vi "CRYLast curve or result read.vi"(8 "Extension":string="Result          ", 11 "Filepath":path) -> (0 "Error":bool, 3 "Flat Data or Result":string)   [LabVIEW 2013]
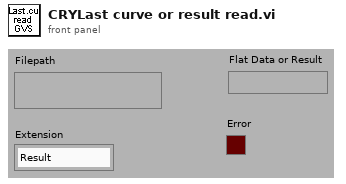
[diagram p1: front panel]
types:
  T1 = enum16{"read/write", "read-only", "write-only", "write-only (truncate)"}
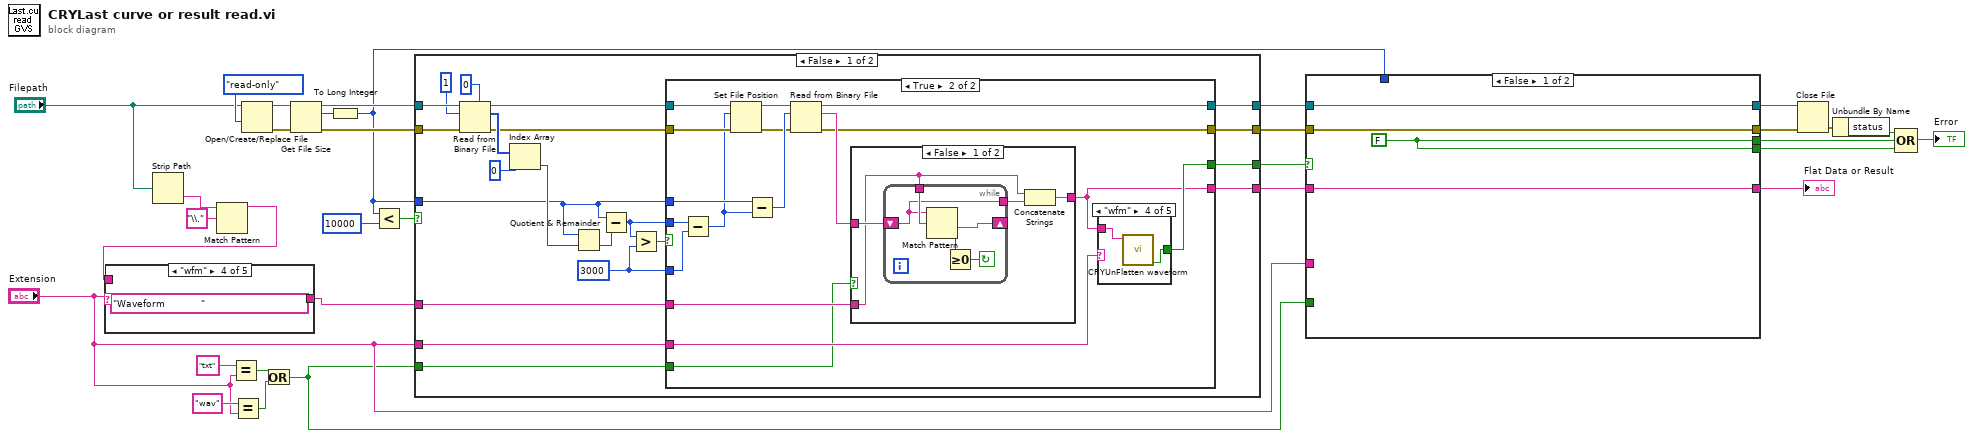
[diagram p0: block diagram]
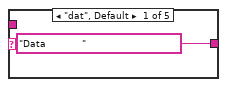
[diagram p2: hidden frame]
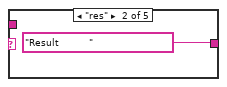
[diagram p3: hidden frame]
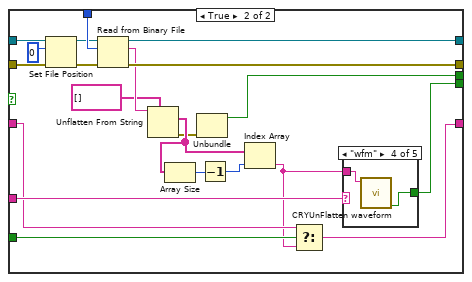
[diagram p6: hidden frame]
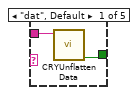
[diagram p7: hidden frame]
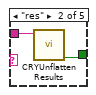
[diagram p8: hidden frame]
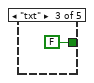
[diagram p9: hidden frame]
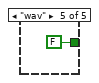
[diagram p10: hidden frame]
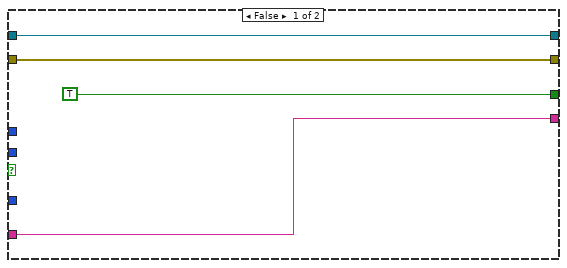
[diagram p11: hidden frame]
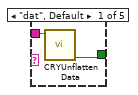
[diagram p13: hidden frame]
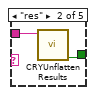
[diagram p14: hidden frame]
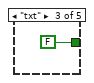
[diagram p15: hidden frame]
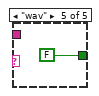
[diagram p16: hidden frame]
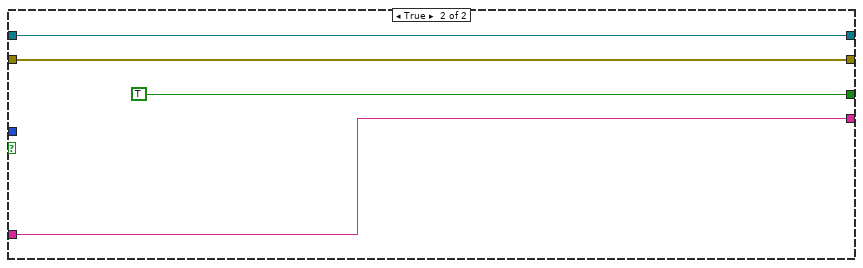
[diagram p17: hidden frame]
diagram:
  n1 = Strip Path(path="Filepath") -> (name=w9:string)  [unwired: 1 out]
  n2 = Match Pattern(string=w9, regular expression="\\.") -> (before substring=w7:string)  [unwired: 1 in, 3 out]
  n3 = case shown="\"wfm\"" "Extension" {
    tunnel: ["Data            " "Result          " w35 "Waveform            " w37] -> w11
    tunnel: w7 -> [_ _ w35 _ w37]
    frame "dat", Default {
    }
    frame "res" {
    }
    frame "txt" {
    }
    frame "wfm" {
    }
    frame "wav" {
    }
  }
  n4 = Equal?(x="txt", y="Extension") -> (x = y?=w5:bool)
  n5 = Equal?(x="wav", y="Extension") -> (x = y?=w6:bool)
  n6 = Open/Create/Replace File(file path (use dialog)="Filepath", access (0:read/write)=T1."read-only" ("open mode (0)")) -> (refnum out=w32:refnum<file>, error out=w31:errorcluster)  [unwired: 1 in, 4 out]
  n7 = Or(x=w5, y=w6) -> (x .or. y?=w1:bool)
  n8 = Get File Size(file=w32, error in=w31) -> (refnum out=w21:refnum<file>, size (in bytes)=w12:i64, 0:w20:errorcluster)
  n9 = To Long Integer(number=w12) -> (32bit integer=w15:i32)
  n10 = Less?(x=w15, y=10000 ("offset")) -> (x < y?=w22:bool)
  n11 = case shown="False" w22 {
    tunnel: w21 -> [w58 w100]
    tunnel: w20 -> [w57 w99]
    tunnel: w15 -> [w41 _]
    tunnel: [w45 TRUE ("Error?")] -> w19
    tunnel: [w44 w98] -> w18
    tunnel: [w43 w99] -> w17
    tunnel: [w42 w100] -> w16
    tunnel: w11 -> [w40 w98]
    tunnel: "Extension" -> [w39 _]
    tunnel: w1 -> [w38 _]
    frame False {
      w48 = 3000 ("y")
      n12 = Read from Binary File(5:0 ("count"), 8:w57, 10:1 ("count"), 11:w58) -> (0:w46:errorcluster, 2:w54:i32[], 3:w47:refnum<file>)  [unwired: 3 out]
      n13 = Index Array(array=w54, index=0 ("Index")) -> (element=w52:i32)
      n14 = Quotient & Remainder(x=w41, y=w52) -> (floor(x/y)=w51:i32)  [unwired: 1 out]
      n15 = Subtract(x=w41, y=w51) -> (x-y=w49:i32)
      n16 = Greater?(x=w49, y=w48) -> (0:w50:bool)
      n17 = case shown="True" w50 {
        tunnel: w49 -> [_ w79]
        tunnel: w48 -> [_ w78]
        tunnel: w47 -> [w61 w77]
        tunnel: w46 -> [w60 w76]
        tunnel: [TRUE ("Error?") w74] -> w45
        tunnel: [w59 w68] -> w44
        tunnel: [w60 w73] -> w43
        tunnel: [w61 w72] -> w42
        tunnel: w41 -> [_ w71]
        tunnel: w40 -> [w59 w67]
        tunnel: w39 -> [_ w64]
        tunnel: w38 -> [_ w63]
        frame False {
        }
        frame True {
          n18 = Subtract(x=w79, y=w78) -> (x-y=w70:i32)
          n19 = Set File Position(offset (in bytes) (0)=w70, refnum=w77, error in=w76) -> (refnum out=w66:refnum<file>, error out=w65:errorcluster)  [unwired: 1 out]
          n20 = Subtract(x=w71, y=w70) -> (x-y=w69:i32)
          n21 = Read from Binary File(8:w65, 10:w69, 11:w66) -> (0:w73:errorcluster, 2:w75:string, 3:w72:refnum<file>)  [unwired: 4 out]
          n22 = case shown="False" w63 {
            tunnel: w75 -> [w83 _]
            tunnel: [w81 w89] -> w68
            tunnel: w67 -> [w80 w89]
            frame False {
              n23 = while {
                tunnel: [w84] -> w82
                tunnel: w80 -> [w88]
                shift-left: w83 -> [w84]
                shift-right: [w87] -> _
                stop <- w85 continue-if-true
                n24 = Match Pattern(string=w84, regular expression=w88) -> (after substring=w87:string, offset past match=w86:i32)  [unwired: 3 out]
                n25 = Greater Or Equal To 0?(x=w86) -> (x >= 0?=w85:bool)
              }
              n26 = Concatenate Strings(w80, w82) -> (w81:string)
            }
            frame True {
            }
          }
          n27 = case shown="\"wfm\"" w64 {
            tunnel: [w91 w92 FALSE ("Error?") w95 FALSE ("Error?")] -> w74
            tunnel: w68 -> [w90 w93 _ w96 _]
            frame "dat", Default {
              n28 = call "CRYUnflatten Data.vi"("Unflatten data"=w90) -> ("Error?"=w91:bool)  [unwired: 8 in, 2 out]
            }
            frame "res" {
              n29 = call "CRYUnflatten Results.vi"("Unflatten Result"=w93) -> ("Error?"=w92:bool)  [unwired: 8 in, 2 out]
            }
            frame "txt" {
            }
            frame "wfm" {
              n30 = call "CRYUnFlatten waveform.vi"("Unflatten Waveform"=w96) -> ("Error?"=w95:bool)  [unwired: 8 in, 2 out]
            }
            frame "wav" {
            }
          }
        }
      }
    }
    frame True {
    }
  }
  n31 = case shown="False" w19 {
    tunnel: [w103 w126] -> w30
    tunnel: [w104 w125] -> w29
    tunnel: [w102 w110] -> w27
    tunnel: [w102 w123] -> w25
    tunnel: [w105 w106] -> w13
    tunnel: w18 -> [w105 w108]
    tunnel: w17 -> [w103 w117]
    tunnel: w16 -> [w104 w116]
    tunnel: w15 -> [_ w115]
    tunnel: "Extension" -> [_ w111]
    tunnel: w1 -> [_ w109]
    frame False {
      w102 = FALSE ("err")
    }
    frame True {
      n32 = Set File Position(offset (in bytes) (0)=0 ("pos offset (0)"), refnum=w116, error in=w117) -> (refnum out=w113:refnum<file>, error out=w112:errorcluster)  [unwired: 1 out]
      n33 = Read from Binary File(8:w112, 10:w115, 11:w113) -> (0:w126:errorcluster, 2:w124:string, 3:w125:refnum<file>)  [unwired: 4 out]
      n34 = Unflatten From String(type=string[] [], binary string=w124) -> (value=w121:string[], error out=w114:errorcluster)  [unwired: 1 in, 3 out]
      n35 = Array Size(array=w121) -> (size(s)=w120:i32)
      n36 = Unbundle(w114) -> ("status"=w123:bool)  [unwired: 2 out]
      n37 = Decrement(x=w120) -> (x-1=w119:i32)
      n38 = Index Array(array=w121, index=w119) -> (element=w107:string)
      n39 = Select(t=w108, s=w109, f=w107) -> (s? t:f=w106:string)
      n40 = case shown="\"wfm\"" w111 {
        tunnel: [w128 w129 FALSE ("Error?") w132 FALSE ("Error?")] -> w110
        tunnel: w107 -> [w127 w130 _ w133 _]
        frame "dat", Default {
          n41 = call "CRYUnflatten Data.vi"("Unflatten data"=w127) -> ("Error?"=w128:bool)  [unwired: 8 in, 2 out]
        }
        frame "res" {
          n42 = call "CRYUnflatten Results.vi"("Unflatten Result"=w130) -> ("Error?"=w129:bool)  [unwired: 8 in, 2 out]
        }
        frame "txt" {
        }
        frame "wfm" {
          n43 = call "CRYUnFlatten waveform.vi"("Unflatten Waveform"=w133) -> ("Error?"=w132:bool)  [unwired: 8 in, 2 out]
        }
        frame "wav" {
        }
      }
    }
  }
  "Flat Data or Result" <- w13
  n44 = Close File(refnum=w29, error in=w30) -> (error out=w28:errorcluster)  [unwired: 1 out]
  n45 = Unbundle By Name(w28) -> ("status"=w26:bool)
  n46 = Compound Arithmetic op=OR(w26, w25, w27) -> (→"Error":bool)
